vi "Save image.vi"(8 "error in (no error)":errorcluster, 9 "Base name":path=path "Image_", 10 "Path":path, 11 "Image in":T1) -> (0 "error out":errorcluster, 3 "Image out":T1)   [LabVIEW 2020]
uses:
  <vilib>/vision/Image Controls.llb/IMAQ Image.ctl
  controls/FGV actions -- enum.ctl
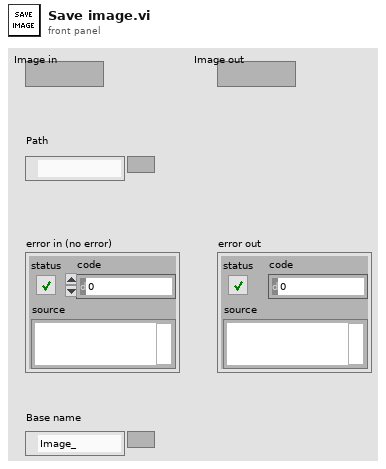
[diagram p1: front panel]
types:
  T1 = typedef "IMAQ Image.ctl" = refnum<image>
  T2 = typedef "FGV actions -- enum.ctl" = enum16{"Reset", "Get", "Increment"}
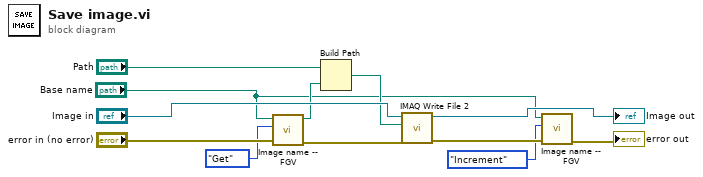
[diagram p0: block diagram]
diagram:
  n1 = call "Image name -- FGV.vi"("error in (no error)"="error in (no error)", "Action"=FGV_actions_--_enum."Get", "Base name"="Base name") -> ("error out"=w6:errorcluster, "Path out"=w9:path)  [unwired: 7 in]
  n2 = Build Path(base path="Path", name or relative path=w9) -> (appended path=w8:path)
  n3 = call-poly "IMAQ Write File 2"("error in (no error)"=w6, "File Path"=w8, "Image"="Image in") -> ("error out"=w5:errorcluster, "Image Out (duplicate)"=→"Image out":T1)  [unwired: 7 in]
  n4 = call "Image name -- FGV.vi"("error in (no error)"=w5, "Action"=FGV_actions_--_enum."Increment", "Base name"="Base name") -> ("error out"=→"error out":errorcluster)  [unwired: 7 in, 1 out]
